vi "Read Created At.vi"(8 "error in (no error)":errorcluster, 11 "Oauth2.GitLab in":refnum<class "Oauth2.GitLab.lvclass">) -> (0 "error out":errorcluster, 2 "Created At":u32, 3 "Oauth2.GitLab out":refnum<class "Oauth2.GitLab.lvclass">)   [LabVIEW 2020, in "Oauth2.GitLab.lvclass"]
uses:
  Oauth2.GitLab.lvclass
  C:/Data/1_Projects/CIGH_Oauth2/source/Oauth2/Oauth2.lvclass
  Oauth2/Oauth2.lvclass
  OAuthToken/OAuth2 Token Element -- enum.ctl
  OAuthToken/OAuthAccessToken.lvclass
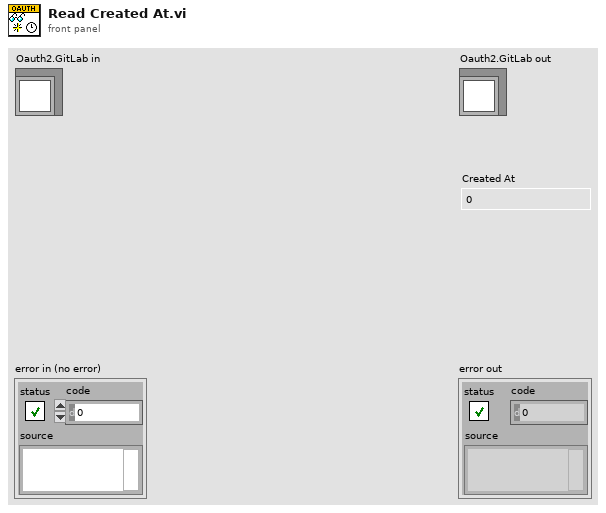
[diagram p1: front panel]
types:
  T1 = typedef "OAuthAccessToken.lvclass/OAuth2 Token Element -- enum.ctl" = enum16{"client_id", "client_secret", "response_type", "scope", "redirect_uri", "error", "error_description", "error_uri", "grant_type", "code", "access_token", "token_type", "expires_in", "username", "password", "refresh_token", "code_challenge", "code_challenge_method", "reverse_proxy_uri", "endpoint element"}
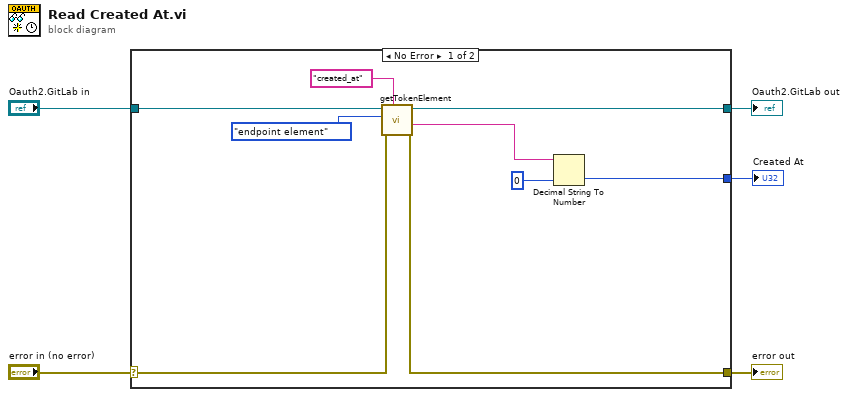
[diagram p0: block diagram]
diagram:
  n1 = case shown="No Error" "error in (no error)" {
    selector: "error in (no error)" -> [w10 w16]
    tunnel: [w9 w16] -> w4
    tunnel: [w13 w15] -> w2
    tunnel: "Oauth2.GitLab in" -> [w14 w15]
    tunnel: [w6 _] -> w1
    frame No Error {
      n2 = call "getTokenElement.vi"("Endpoint Element Name"="created_at", "error in (no error)"=w10, "Token element"=OAuth2_Token_Element_--_enum."endpoint element", "Oauth2 in"=w14) -> ("error out"=w9:errorcluster, "Value"=w8:string, "Oauth2 out"=w13:refnum<class "Oauth2.GitLab.lvclass">)  [unwired: 3 in, 2 out]
      n3 = Decimal String To Number(string=w8, default (0L)=u32 0) -> (number=w6:u32)  [unwired: 1 in, 1 out]
    }
    frame Error {
    }
  }
  "error out" <- w4
  "Oauth2.GitLab out" <- w2
  "Created At" <- w1
